vi "solar Handshake.vi"(8 "error in (no error)":errorcluster, 9 "TLM_DATA":variant, 10 "TLM":string, 11 "solar in":refnum<class "solar.lvclass">) -> (0 "error out":errorcluster, 3 "solar out":refnum<class "solar.lvclass">)   [LabVIEW 2018, in "solar.lvclass"]
doc: "This handles the handshaking between local and remote target. Specify the telemetry and data to return to COSMOS and the calling target. This returns the local handshake before sending the Voyager telemetry and handshake then broadcasts the telemetry to all subscribed targets. Lastly the telemetry is logged if defined."
uses:
  solar.lvclass
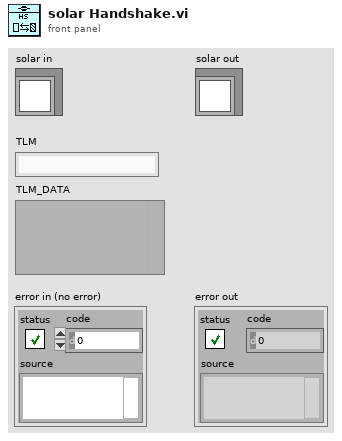
[diagram p1: front panel]
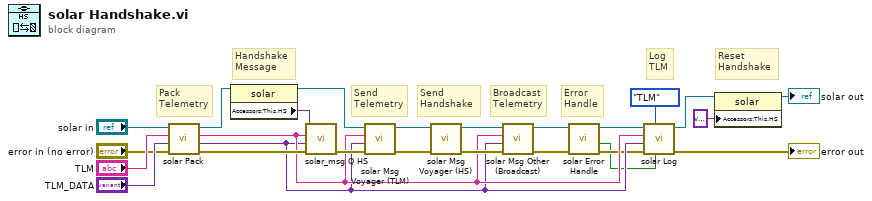
[diagram p0: block diagram]
diagram:
  # "Error\nHandle"
  # "Send\nHandshake"
  # "Log\nTLM"
  # "Send\nTelemetry"
  # "Handshake\nMessage"
  # "Pack\nTelemetry"
  # "Reset\nHandshake"
  # "Broadcast\nTelemetry"
  n1 = call-dynamic "solar Pack.vi"("error in (no error)"="error in (no error)", "TLM_DATA in"="TLM_DATA", "TLM in"="TLM", "solar in"="solar in") -> ("error out"=w17:errorcluster, "TLM_DATA out"=w7:variant, "TLM out"=w8:string, "solar out"=w16:refnum<class "solar.lvclass">)  [unwired: 4 in]
  n2 = property class="solar"(reference=w16) -> (reference out=w14:refnum<class "solar.lvclass">, "Accessors:This.HS"=w15:variant)  [unwired: 1 in, 1 out]
  n3 = call "solar_msg Q HS.vi"("error in (no error)"=w17, "TLM_DATA"=w7, "TLM"=w8, "CMD_DATA ('HS' Attr)"=w15) -> ("error out"=w11:errorcluster)  [unwired: 7 in]
  n4 = call "solar Msg Voyager (TLM).vi"("error in (no error)"=w11, "TLM_DATA (No HDR)"=w7, "TLM"=w8, "solar in"=w14) -> ("error out"=w13:errorcluster, "solar out"=w12:refnum<class "solar.lvclass">)  [unwired: 6 in]
  n5 = call "solar Msg Voyager (HS).vi"("error in (no error)"=w13, "solar in"=w12) -> ("error out"=w10:errorcluster, "solar out"=w9:refnum<class "solar.lvclass">)  [unwired: 8 in]
  n6 = call "solar Msg Other (Broadcast).vi"("error in (no error)"=w10, "TLM_DATA"=w7, "TLM"=w8, "solar in"=w9) -> ("error out"=w3:errorcluster, "solar out"=w5:refnum<class "solar.lvclass">)  [unwired: 6 in]
  n7 = call-dynamic "solar Error Handle.vi"("error in (no error)"=w3, "solar in"=w5) -> ("error out"=w2:errorcluster, "Clear Error?"=w1:bool, "solar out"=w4:refnum<class "solar.lvclass">)  [unwired: 7 in]
  n8 = call "solar Log.vi"("Clear Error? (T)"=w1, "Type (TLM)"=enum8{"CMD", "TLM"}."TLM", "error in (no error)"=w2, "DATA"=w7, "MSG"=w8, "solar in"=w4) -> ("error out"=→"error out":errorcluster, "solar out"=w22:refnum<class "solar.lvclass">)  [unwired: 4 in]
  n9 = property class="solar"(reference=w22, "Accessors:This.HS"=variant ("This:Handshake")) -> (reference out=→"solar out":refnum<class "solar.lvclass">)  [unwired: 1 in, 1 out]
